vi "Name Value Write Tags.vi"(0 "File Path":path, 7 "Tags Group Array":string[][](array[string]), 11 "Error In":errorcluster) -> (15 "Error Out":errorcluster)   [LabVIEW 2020]
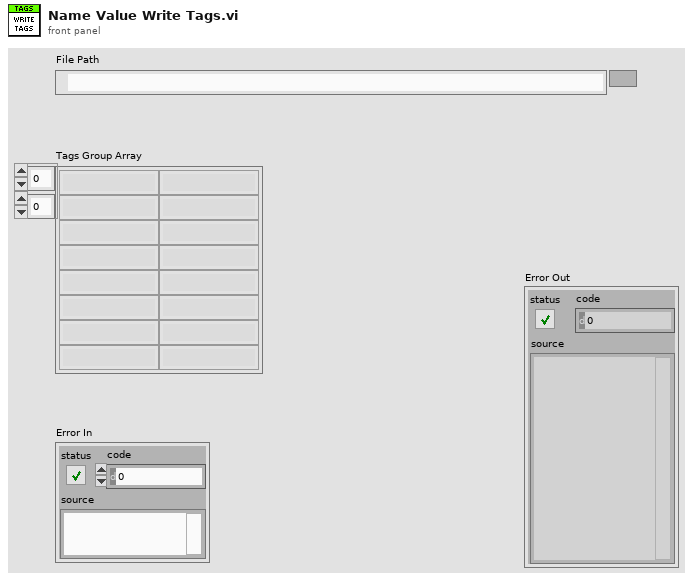
[diagram p1: front panel]
types:
  T1 = enum16{"open", "replace", "create", "open or create", "replace or create", "replace or create with confirmation"}
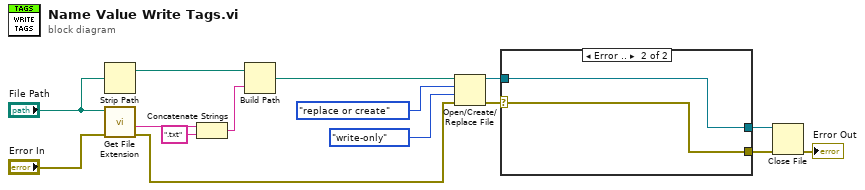
[diagram p0: block diagram]
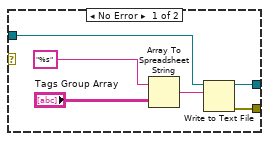
[diagram p2: hidden frame]
diagram:
  n1 = Strip Path(path="File Path") -> (stripped path=w5:path)  [unwired: 1 out]
  n2 = call <vilib>:"Get File Extension.vi"("error in (no error)"="Error In", "file"="File Path") -> ("error out"=w2:errorcluster, "filename without extension"=w7:string)  [unwired: 5 in, 3 out]
  n3 = Concatenate Strings(w7, ".txt" ("string")) -> (w4:string)
  n4 = Build Path(base path=w5, name or relative path=w4) -> (appended path=w1:path)
  n5 = Open/Create/Replace File(file path (use dialog)=w1, error in=w2, operation (0:open)=T1."replace or create", access (0:read/write)=enum16{"read/write", "read-only", "write-only"}."write-only") -> (refnum out=w15:refnum<file>, error out=w12:errorcluster)  [unwired: 2 in, 1 out]
  n6 = case shown="Error .." w12 {
    selector: w12 -> [_ w22]
    tunnel: w15 -> [w19 w23]
    tunnel: [w18 w23] -> w11
    tunnel: [w16 w22] -> w10
    frame No Error {
      n7 = Array To Spreadsheet String(array="Tags Group Array", 3:"%s") -> (spreadsheet string=w20:string)  [unwired: 1 in]
      n8 = Write to Text File(file (use dialog)=w19, text=w20) -> (refnum out=w18:refnum<file>, error out=w16:errorcluster)  [unwired: 2 in, 1 out]
    }
    frame Error {
    }
  }
  n9 = Close File(refnum=w11, error in=w10) -> (error out=→"Error Out":errorcluster)  [unwired: 1 out]
